vi "Clean up volume table.vi"(8 "error in (no error)":errorcluster, 10 "Volume table in":dbl[][](array[numeric]), 11 "Tomo in":refnum<class "Tomo.lvclass">) -> (0 "error out":errorcluster, 2 "Volume table out":dbl[][](array[numeric]), 3 "Tomo out":refnum<class "Tomo.lvclass">)   [LabVIEW 2012, in "Tomo.lvclass"]
uses:
  Tomo.lvclass
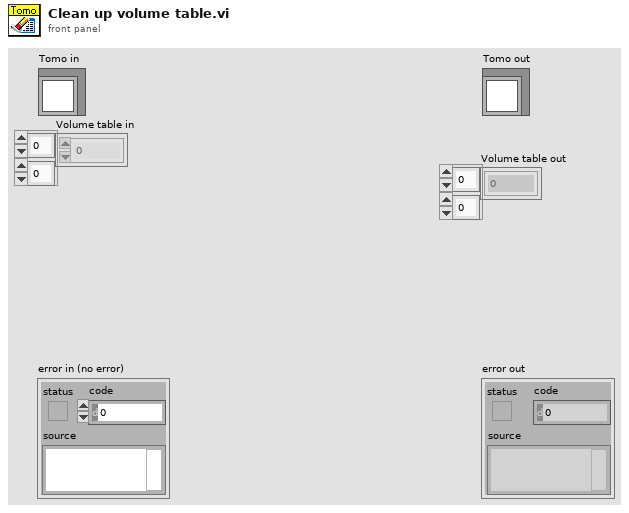
[diagram p1: front panel]
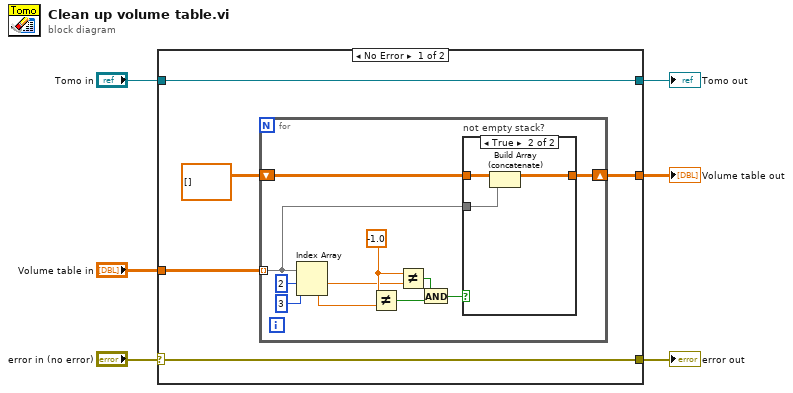
[diagram p0: block diagram]
diagram:
  n1 = case shown="No Error" "error in (no error)" {
    selector: "error in (no error)" -> [w10 w28]
    tunnel: [w10 w28] -> w5
    tunnel: [w11 w27] -> w3
    tunnel: "Tomo in" -> [w11 w27]
    tunnel: "Volume table in" -> [w9 _]
    tunnel: [w7 _] -> w1
    frame No Error {
      n2 = for {
        tunnel: w9 -> [w15] mode=indexing
        shift-right: [w16] -> w7
        shift-left: dbl[][] [] ("Volume table in") -> [w17]
        w14 = -1.0
        n3 = Index Array(array=w15, index #1=2 ("index"), index #2=3 ("index")) -> (element #1=w13:dbl, element #2=w12:dbl)
        n4 = Not Equal?(x=w14, y=w12) -> (x != y?=w20:bool)
        n5 = Not Equal?(x=w14, y=w13) -> (x != y?=w19:bool)
        n6 = And(x=w19, y=w20) -> (x .and. y?=w18:bool)
        n7 = case "not empty stack?" shown="True" w18 {
          tunnel: w17 -> [w23 w26]
          tunnel: [w23 w24] -> w16
          tunnel: w15 -> [_ w25]
          frame False {
          }
          frame True {
            n8 = Build Array (concatenate)(w26, w25) -> (w24:dbl[][])
          }
        }
      }
    }
    frame Error {
    }
  }
  "error out" <- w5
  "Tomo out" <- w3
  "Volume table out" <- w1
